vi "CRYGet Channel Index from OpendArray.vi"(11 "Channel Name":string) -> (3 "index of Channel":i32=-1)   [LabVIEW 2013]
uses:
  CRYMisc vis settings global.vi
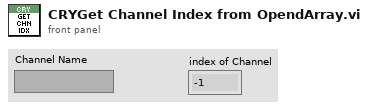
[diagram p1: front panel]
types:
  T1 = cluster{"Chn Name":string, "Count":i16, "Opend Idx":i16}[]
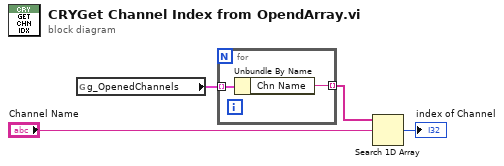
[diagram p0: block diagram]
diagram:
  n1 = global read "CRYMisc vis settings global.vi" "g_OpenedChannels"() -> (w4:T1)
  n2 = for {
    tunnel: w4 -> [w6] mode=indexing
    tunnel: [w5] -> w3 mode=indexing
    n3 = Unbundle By Name(w6) -> ("Chn Name"=w5:string)
  }
  n4 = Search 1D Array(1D array=w3, element="Channel Name") -> (index of element=→"index of Channel":i32)  [unwired: 1 in]
